vi "ExampleRGBAImageData.vi"(1 "Image Size":T2={"Width"=256, "Height"=128}) -> (0 "RGB Image Data":T1)   [LabVIEW 2020, in "g_ar_toolkit.test.lvlib" / "Image.lvclass"]
uses:
  Image.lvclass
  g_ar_toolkit/Image Size Cluster.ctl
  Image.lvclass/Image.ctl
  g_ar_toolkit.lvlib
  <vilib>/picture/picture.llb/imagedata.ctl
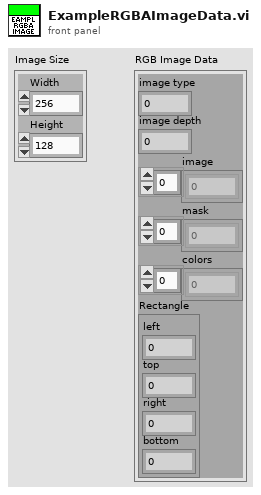
[diagram p1: front panel]
types:
  T1 = typedef "imagedata.ctl" = cluster{"image type":i32, "image depth":i32, "image":u8[], "mask":u8[], "colors":u32[], "Rectangle":cluster{"left":i16, "top":i16, "right":i16, "bottom":i16}}
  T2 = typedef "g_ar_toolkit.lvlib/Image Size Cluster.ctl" = cluster{"Width":u16, "Height":u16}
  T3 = cluster{"left":i16, "top":i16, "right":i16, "bottom":i16}
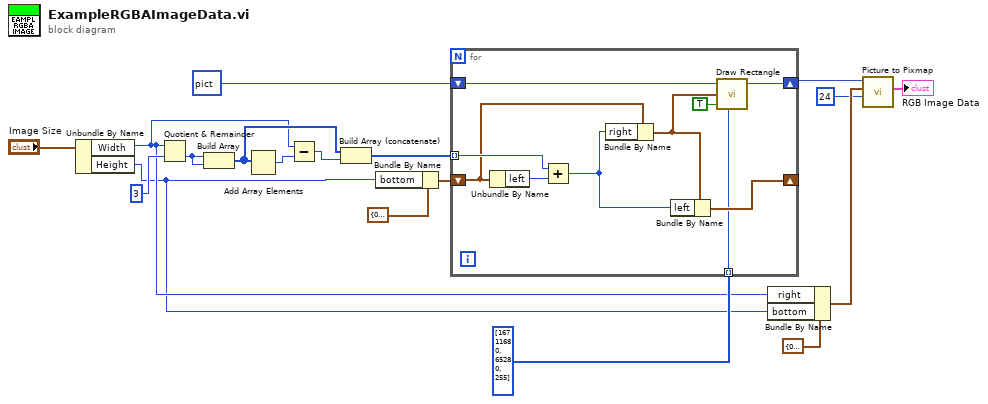
[diagram p0: block diagram]
diagram:
  n1 = Unbundle By Name("Image Size") -> ("Width"=w4:u16, "Height"=w3:u16)
  n2 = Quotient & Remainder(x=w4, y=u16 3) -> (floor(x/y)=w15:u16)  [unwired: 1 out]
  n3 = Build Array(w15, w15) -> (w12:u16[])
  n4 = Add Array Elements(numeric array=w12) -> (sum=w14:u16)
  n5 = Subtract(x=w4, y=w14) -> (x-y=w13:u16)
  n6 = Build Array (concatenate)(w12, w13) -> (w11:u16[])
  n7 = Bundle By Name(cluster=T3 {"left"=0, "top"=0, "right"=0, "bottom"=0} ("rect"), "bottom"=w3) -> (w9:T3)
  n8 = for {
    shift-right: [w21] -> w7
    shift-left: picture data[5B] ("picture") -> [w28]
    tunnel: w11 -> [w26] mode=indexing
    shift-right: [w22] -> _
    shift-left: w9 -> [w25]
    tunnel: u32[] [16711680, 65280, 255] ("color(black)") -> [w19] mode=indexing
    n9 = Unbundle By Name(w25) -> ("left"=w27:i16)
    n10 = Add(x=w26, y=w27) -> (x+y=w23:u16)
    n11 = Bundle By Name(cluster=w25, "right"=w23) -> (w24:T3)
    n12 = Bundle By Name(cluster=w24, "left"=w23) -> (w22:T3)
    n13 = call <vilib>:"Draw Rectangle.vi"("picture"=w28, "rect"=w24, "fill?(F)"=TRUE, "color(black)"=w19) -> ("new picture"=w21:picture)  [unwired: 5 in]
  }
  n14 = Bundle By Name(cluster=T3 {"left"=0, "top"=0, "right"=0, "bottom"=0} ("rect"), "right"=w4, "bottom"=w3) -> (w5:T3)
  n15 = call <vilib>:"Picture to Pixmap.vi"("depth"=24, "rect"=w5, "picture"=w7) -> ("image data"=→"RGB Image Data":T1)  [unwired: 7 in, 1 out]
